vi "Test Client.vi"() -> ()   [LabVIEW 2016, in "Instrument.Example.lvclass"]
uses:
  Instrument.Example.lvclass
  <userlib>/LevyLab/Levylab Instruments/SMOs/RemoteControl.STM/RemoteControl.STM.lvclass
  C:/Program Files (x86)/National Instruments/LabVIEW 2016/user.lib/LevyLab/Levylab Instruments/SMOs/RemoteControl/RemoteControl.lvclass
  <userlib>/_OpenG.lib/numeric/numeric.llb/Random Number Within Range - DBL__ogtk.vi
  <userlib>/LevyLab/Levylab Instruments/SMOs/RemoteControl/RemoteControl.lvclass
panel:
  out "Data out":variant
  out "Command out":string
  out "Numeric":i32
  in  "stop":bool
  out "Waveform Chart":u32(graph)
  out "error out":errorcluster
  out "execution time (ms)":u32
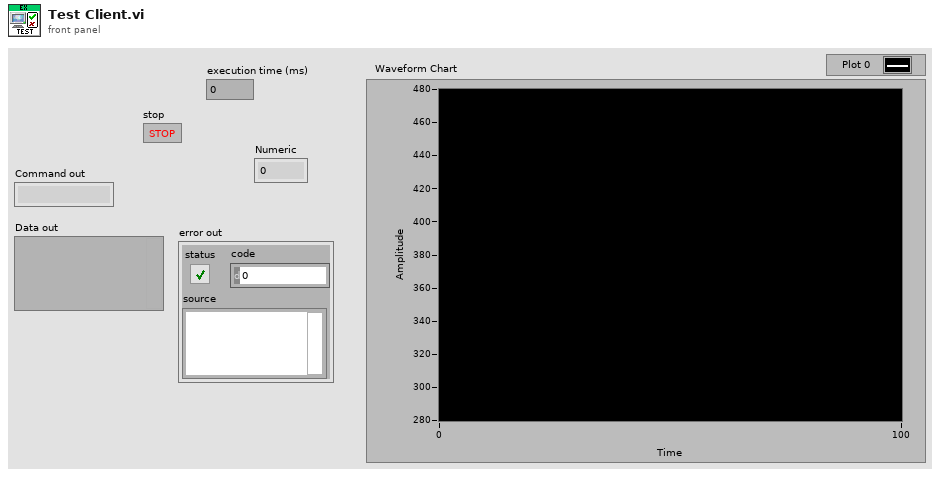
[diagram p1: front panel]
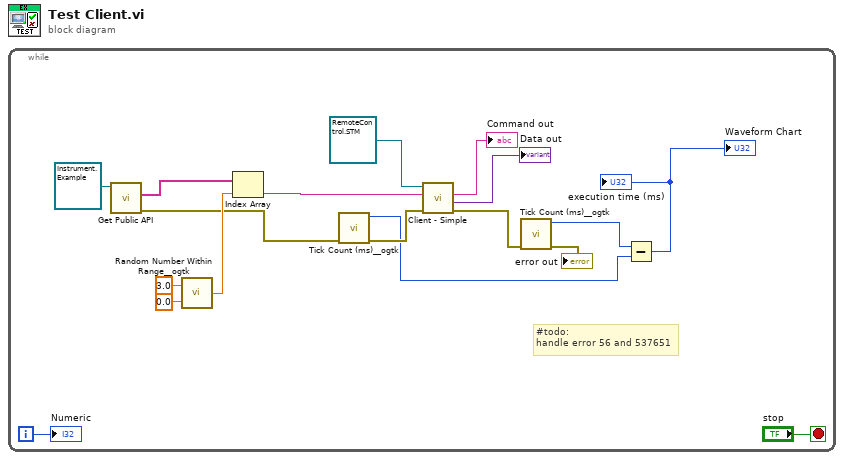
[diagram p0: block diagram]
diagram:
  n1 = while {
    i -> [w14]
    stop <- "stop" stop-if-true
    # "#todo:\nhandle error 56 and 537651"
    n2 = call-dynamic "Get Public API.vi"("Instrument.Example In"=refnum<class "Instrument.Example.lvclass"> refnum ("Instrument.SR7270 in")) -> ("error out"=w7:errorcluster, "Commands"=w12:string[])  [unwired: 8 in, 1 out]
    n3 = call-poly <userlib>:"Random Number Within Range__ogtk.vi"("High"=3.0, "Low"=0.0) -> ("Random Number"=w16:dbl)  [unwired: 3 in]
    n4 = Index Array(array=w12, index=w16) -> (element=w11:string)
    n5 = call <userlib>:"Tick Count (ms)__ogtk.vi"("error in (no error)"=w7) -> ("error out"=w6:errorcluster, "millisecond timer value"=w2:u32)  [unwired: 9 in]
    n6 = call <userlib>:"Client - Simple.vi"("error in (no error)"=w6, "Command"=w11, "RemoteControl in"=refnum<class "RemoteControl.STM.lvclass"> refnum ("RemoteControl.STM in")) -> ("error out"=w5:errorcluster, "Data out"=→"Data out":variant, "Command out"=→"Command out":string)  [unwired: 5 in, 1 out]
    n7 = call <userlib>:"Tick Count (ms)__ogtk.vi"("error in (no error)"=w5) -> ("error out"=→"error out":errorcluster, "millisecond timer value"=w3:u32)  [unwired: 9 in]
    n8 = Subtract(x=w3, y=w2) -> (x-y=→"execution time (ms)" →"Waveform Chart":u32)
    "Numeric" <- w14
  }
